vi "PR Enable Acquire Signal.vi"(0 "bEnabled":bool) -> ()   [LabVIEW 2022 SP3, in "BS6006PRPLUS.lvlib"]
doc: "The function sets the status of the function of the analog-to-digital converter of pulser/receiver.\n\nextern \"C\" BS6006PRPLUS_API void __cdecl PR_EnableAcquireSignal(bool bEnabled);"
uses:
  BS6006PRPLUS.lvlib
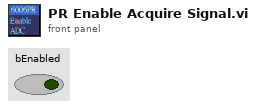
[diagram p1: front panel]
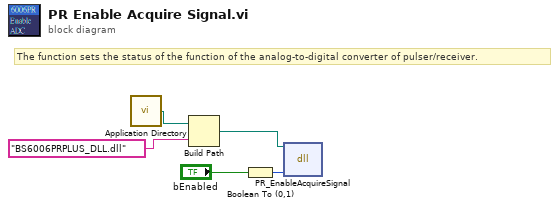
[diagram p0: block diagram]
diagram:
  # "The function sets the status of the function of the analog-to-digital converter of pulser/receiver."
  n1 = call <vilib>:"Application Directory.vi"() -> ("Application Directory"=w3:path)
  n2 = Build Path(base path=w3, name or relative path="BS6006PRPLUS_DLL.dll") -> (appended path=w1:path)
  n3 = Boolean To (0,1)(Boolean="bEnabled") -> (0, 1=w4:i16)
  n4 = dll-call lib="E:/Broadsound_Program/PulserReceiver/6006PR PLUS/API/DLL/LabVIEW 15/VIs/BS6006PRPLUS_DLL.dll" fn="PR_EnableAcquireSignal"(path in=w1, "bEnabled"=w4) -> ()  [unwired: 4 in, 2 out]
